vi "qSPA_Hex_String.vi"(0 "System no.":i32=1 min=1 max=4 step=1, 2 "Designator to query":string[](array[string]), 3 "Without designators?":bool, 4 "Parameter no. (hex)":u32[](array[numeric]) format="%.0x", 5 "error in":errorcluster) -> (14 "Parameter string":string[](array[string]), 19 "error out":errorcluster)   [LabVIEW 2026]
doc: "Returns parameter strings for queried designators and hex. parameter numbers. See GCS DLL manual for available parameter numbers. For axis-related parameters, Designator to query is the axis name; for piezo- or sensor-related parameters, the channel number, otherwise a parameter-related one. If \"Without designators?\" is TRUE, all available parameters for all designators are returned. For parameter numbers which output a numerical value use SPA?_hex.vi.\nOld VI - please use SPA?.vi instead.\n\nE-710: Use HPA?.vi to get valid parameter numbers."
uses:
  Communication/Global1.vi
panel:
  # "Returns parameter strings for queried designators and hex. parameter numbers. Old VI - please use \nSPA?.vi instead."
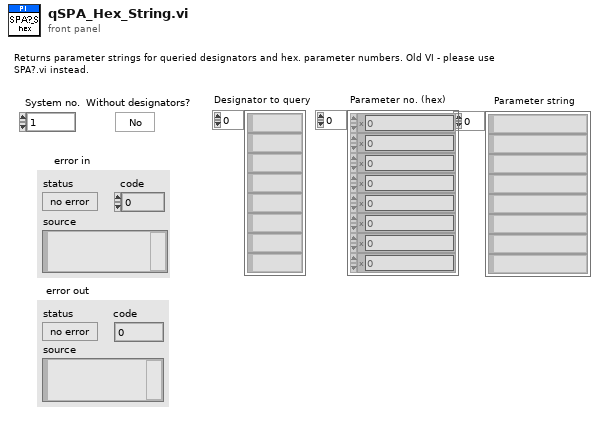
[diagram p1: front panel]
types:
  T1 = enum16{"Disable error check", "Force error check", "Use global settings"}
  T2 = typedef "Syntax.ctl" = enum16{"GCS 1.0", "GCS 2.0", "GCS 3.0"}
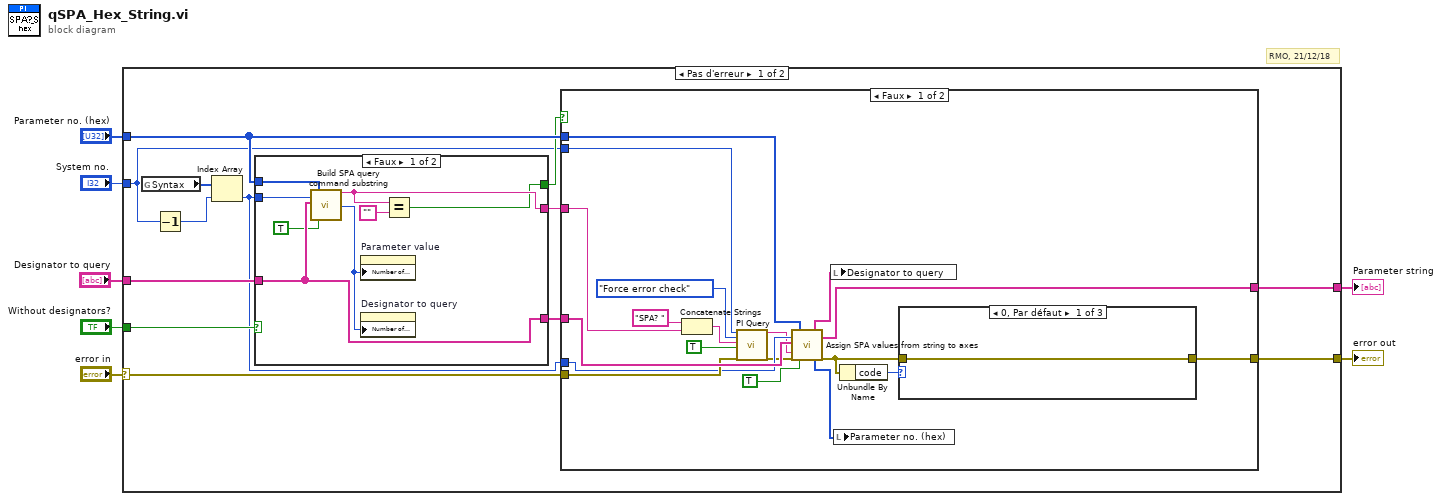
[diagram p0: block diagram]
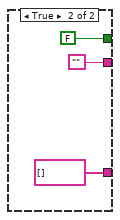
[diagram p2: hidden frame]
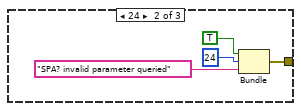
[diagram p3: hidden frame]
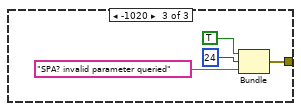
[diagram p4: hidden frame]
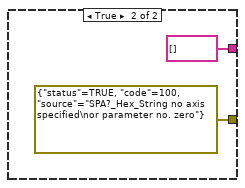
[diagram p5: hidden frame]
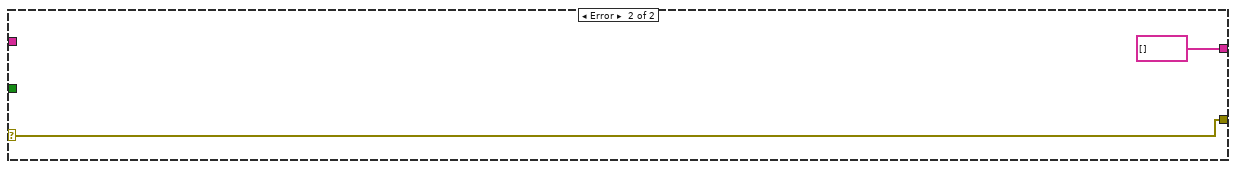
[diagram p6: hidden frame]
diagram:
  # "RMO, 21/12/18"
  n1 = case shown="Pas d'erreur" "error in" {
    selector: "error in" -> [w8 w62]
    tunnel: "Designator to query" -> [w15 _]
    tunnel: "System no." -> [w10 _]
    tunnel: "Parameter no. (hex)" -> [w19 _]
    tunnel: [w18 w62] -> w4
    tunnel: [w16 string[] [] ("Parameter strings")] -> w3
    tunnel: "Without designators?" -> [w14 _]
    frame No Error {
      n2 = global read "Global1.vi" "Syntax"() -> (w11:T2[])
      n3 = Decrement(x=w10) -> (x-1=w12:i32)
      n4 = Index Array(array=w11, index=w12) -> (element=w9:T2)
      n5 = case shown="Faux" w14 {
        tunnel: [w27 "" ("Command substring")] -> w20
        tunnel: w19 -> [w23 _]
        tunnel: [w25 FALSE] -> w17
        tunnel: w15 -> [w24 _]
        tunnel: [w24 string[] [] ("Designator to query")] -> w13
        tunnel: w9 -> [w22 _]
        frame False {
          n6 = call "Build SPA query command substring.vi"("Syntax"=w22, "Axes to query"=w24, "Parameter number (hex)"=w23, "Parameter no. format \n(Decimal: FALSE)"=TRUE ("Parameter no. format \n(Decimal: FALSE)")) -> ("Command substring"=w27:string, "Number of rows"=w26:u32)  [unwired: 1 in, 13 out]
          n7 = property on="Parameter value" class="Tabl (strict)"("Number of Rows"=w26) -> ()  [unwired: 2 in, 2 out]
          n8 = property on="Designator to query" class="Tabl (strict)"("Number of Rows"=w26) -> ()  [unwired: 2 in, 2 out]
          n9 = Equal?(x=w27, y="" ("x")) -> (x = y?=w25:bool)
        }
        frame True {
        }
      }
      n10 = case shown="Faux" w17 {
        tunnel: w8 -> [w44 _]
        tunnel: w20 -> [w47 _]
        tunnel: w13 -> [w46 _]
        tunnel: w10 -> [w41 _]
        tunnel: w19 -> [w40 _]
        tunnel: [w35 errorcluster {"status"=TRUE, "code"=100, "source"="SPA?_Hex_String no axis specified\nor parameter no. zero"} ("error out")] -> w18
        tunnel: [w45 string[] [] ("Parameter strings")] -> w16
        tunnel: w9 -> [w38 _]
        frame False {
          n11 = Concatenate Strings("SPA? ", w47) -> (w48:string)
          n12 = call "PI Query.vi"("System no."=w41, "Error check settings"=T1."Force error check", "String to send"=w48, "Attach termination char.?"=TRUE ("Attach Linefeed?"), "error in"=w44) -> ("String read"=w36:string, "error out"=w37:errorcluster)  [unwired: 2 in, 11 out]
          n13 = call "Assign SPA values from string to axes.vi"("Syntax"=w38, "Queried axes"=w46, "Input string"=w36, "error in"=w37, "Parameter no. (hex)"=w40, "Parameter no. format \n(Decimal: FALSE)"=TRUE ("Parameter no. format \n(Decimal: FALSE)")) -> ("Queried axes out"=w43:string[], "Parameter no. (hex) out"=w42:u32[], "Parameter strings"=w45:string[], "error out"=w33:errorcluster)  [unwired: 1 in, 9 out]
          n14 = local write "Designator to query"(w43) -> ()
          n15 = local write "Parameter no. (hex)"(w42) -> ()
          n16 = Unbundle By Name(w33) -> ("code"=w34:i32)
          n17 = case shown="0, Par défaut" w34 {
            tunnel: [w51 w52 w56] -> w35
            tunnel: w33 -> [w51 _ _]
            frame 0, Default {
            }
            frame 24 {
              n18 = Bundle(TRUE, 24, "SPA? invalid parameter queried") -> (w52:errorcluster)  [unwired: 1 out]
            }
            frame -1020 {
              n19 = Bundle(TRUE, 24, "SPA? invalid parameter queried") -> (w56:errorcluster)  [unwired: 1 out]
            }
          }
        }
        frame True {
        }
      }
    }
    frame Error {
    }
  }
  "error out" <- w4
  "Parameter string" <- w3
